vi "Read Tare.vi"(8 "error in (no error)":errorcluster, 11 "VISA resource name":refnum<visa-resource-name>) -> (0 "error out":errorcluster, 1 "Tare Unit":string, 2 "Tare Value":dbl format="%#.6f", 3 "VISA resource name out":refnum<visa-resource-name>)   [LabVIEW 2017, in "RadWag balances and scales.lvlib"]
doc: "Reads current value of tare."
uses:
  <instrlib>/Prev/RadWag Continuous Read Folder/RadWag balances and scales.lvlib
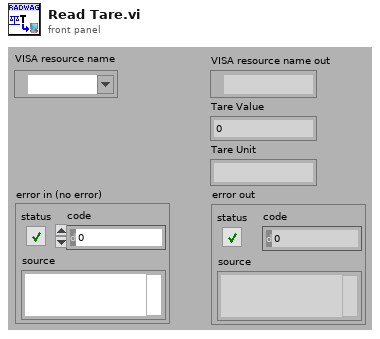
[diagram p1: front panel]
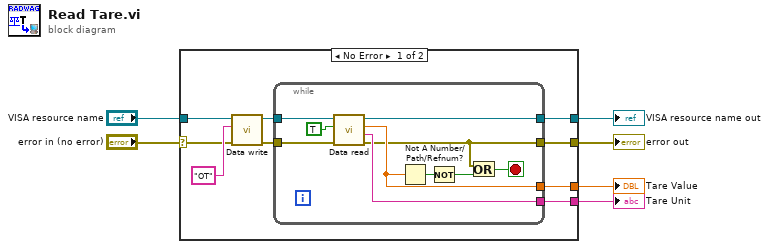
[diagram p0: block diagram]
diagram:
  n1 = case shown="No Error" "error in (no error)" {
    selector: "error in (no error)" -> [w7 w26]
    tunnel: "VISA resource name" -> [w13 w27]
    tunnel: [w11 w26] -> w5
    tunnel: [w10 w27] -> w4
    tunnel: [w9 _] -> w3
    tunnel: [w8 _] -> w2
    frame No Error {
      n2 = call <instrlib>:"Data write.vi"("error in (no error)"=w7, "ID"="OT", "VISA resource name"=w13) -> ("error out"=w12:errorcluster, "VISA resource name out"=w14:refnum<visa-resource-name>)  [unwired: 7 in]
      n3 = while {
        tunnel: w14 -> [w25]
        tunnel: w12 -> [w24]
        tunnel: [w16] -> w11
        tunnel: [w23] -> w10
        tunnel: [w20] -> w9
        tunnel: [w21] -> w8
        stop <- w17 stop-if-true
        n4 = call <instrlib>:"Data read.vi"("error in (no error)"=w24, "Decode Status (F)/ Decode Data (T)"=TRUE ("Status (F)/data(T)"), "VISA resource name"=w25) -> ("error out"=w16:errorcluster, "Unit"=w21:string, "Value"=w20:dbl, "VISA resource name out"=w23:refnum<visa-resource-name>)  [unwired: 2 in, 3 out]
        n5 = Not A Number/Path/Refnum?(number/path/refnum=w20) -> (NaN/Path/Refnum?=w19:bool)
        n6 = Not(x=w19) -> (.not. x?=w18:bool)
        n7 = Or(x=w16, y=w18) -> (x .or. y?=w17:bool)
      }
    }
    frame Error {
    }
  }
  "Tare Value" <- w3
  "VISA resource name out" <- w4
  "error out" <- w5
  "Tare Unit" <- w2
